vi "Read Forces.vi"(8 "error in":errorcluster, 11 "CoreOOB_Rx in":refnum<class "CIFCoreOOB_Rx.lvclass">) -> (0 "error out":errorcluster, 1 "Offset":i32, 2 "Forces":T1[](array[typedef]) {"Force Data" format="%x"}, 3 "CoreOOB_Rx out":refnum<class "CIFCoreOOB_Rx.lvclass">)   [LabVIEW 2021, in "CIFCoreOOB_Rx.lvclass"]
uses:
  CIFCoreOOB_Rx.lvclass
  CIFCoreOOB_Rx.lvclass/CIFCoreOOB_Rx.ctl
  Typedef/Channel Fault Data.ctl
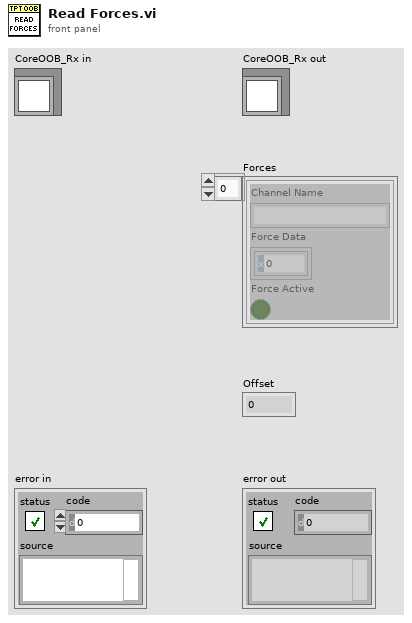
[diagram p1: front panel]
types:
  T1 = typedef "CIFCoreOOB_Rx.lvclass/Channel Fault Data.ctl" = cluster{"Channel Name":string, "Force Data":u8[], "Force Active":bool}
  T2 = typedef "CIFCoreOOB_Rx.lvclass/Template Payload.ctl" = cluster{"Config Data":variant, "Clock Conversion":T3, "Connections":T5[], "Forces":T1[], "FIFO Pub":T6}
  T3 = typedef "Time_CIF_U.lvlib/Clock Conversion Map.ctl" = map{u8, cluster{"Last Reset":i64, "Offset Pair":T4, "Slope":dbl, "1/Slope":dbl}}
  T4 = typedef "Time_CIF_U.lvlib/Timestamp Pair.ctl" = cluster{"System Time":i64, "External Time":i64}
  T5 = typedef "CIFCoreOOB_Rx.lvclass/Channel Connection Data.ctl" = cluster{"Publisher Name":string, "Subscriber Name":string, "Connection Data":u8[]}
  T6 = typedef "CIFCoreOOB_Rx.lvclass/FIFO Publisher.ctl" = cluster{"Publisher Name":string, "New FIFO Instance Config":T7}
  T7 = typedef "ChannelCommon.lvlib/New FIFO Instance Configuration.ctl" = cluster{"Primary":bool, "Backpressure":bool, "Message/FIFO Override":u32}
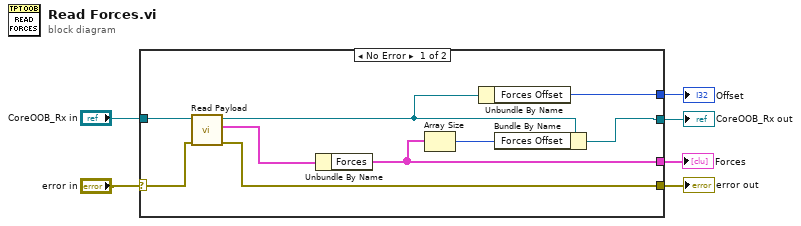
[diagram p0: block diagram]
diagram:
  n1 = case shown="No Error" "error in" {
    selector: "error in" -> [w15 w17]
    tunnel: [w14 w17] -> w6
    tunnel: [w8 w16] -> w5
    tunnel: "CoreOOB_Rx in" -> [w13 w16]
    tunnel: [w7 _] -> w1
    tunnel: [w12 _] -> w2
    frame No Error {
      n2 = call "Read Payload.vi"("error in"=w15, "CoreOOB_Rx in"=w13) -> ("error out"=w14:errorcluster, "data"=w10:T2, "CoreOOB_Rx out"=w9:refnum<class "CIFCoreOOB_Rx.lvclass">)  [unwired: 7 in]
      n3 = Unbundle By Name(w10) -> ("Forces"=w7:T1[])
      n4 = Array Size(array=w7) -> (size(s)=w11:i32)
      n5 = Unbundle By Name(w9) -> ("Forces Offset"=w12:i32)
      n6 = Bundle By Name(cluster=w9, "Forces Offset"=w11) -> (w8:refnum<class "CIFCoreOOB_Rx.lvclass">)
    }
    frame Error {
    }
  }
  "error out" <- w6
  "CoreOOB_Rx out" <- w5
  "Offset" <- w2
  "Forces" <- w1
